vi "Add Key.vi"(6 "value":string, 8 "error in":errorcluster, 9 "key":string, 10 "section":string, 11 "Configuration File in":T1) -> (0 "error out":errorcluster, 3 "Configuration File out":T1)   [LabVIEW 2012, in "configlib.lvlib"]
uses:
  configlib.lvlib
  File Options.ctl
  Configuration File Definition.ctl
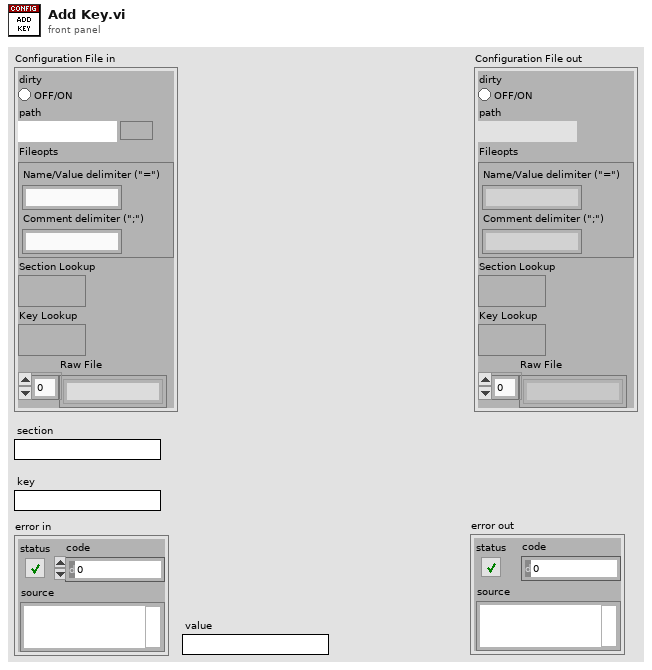
[diagram p1: front panel]
types:
  T1 = typedef "configlib.lvlib/Configuration File Definition.ctl" = cluster{"dirty":bool, "path":path, "Fileopts":T2, "Section Lookup":variant, "Key Lookup":variant, "Raw File":string[]}
  T2 = typedef "configlib.lvlib/File Options.ctl" = cluster{"Name/Value delimiter (\"=\")":string, "Comment delimiter (\";\")":string}
  T3 = typedef "configlib.lvlib/Section Definition.ctl" = cluster{"Keys":string[], "Segments":T4[]}
  T4 = typedef "configlib.lvlib/File Section.ctl" = cluster{"Line Number":i32, "Line Count":i32}
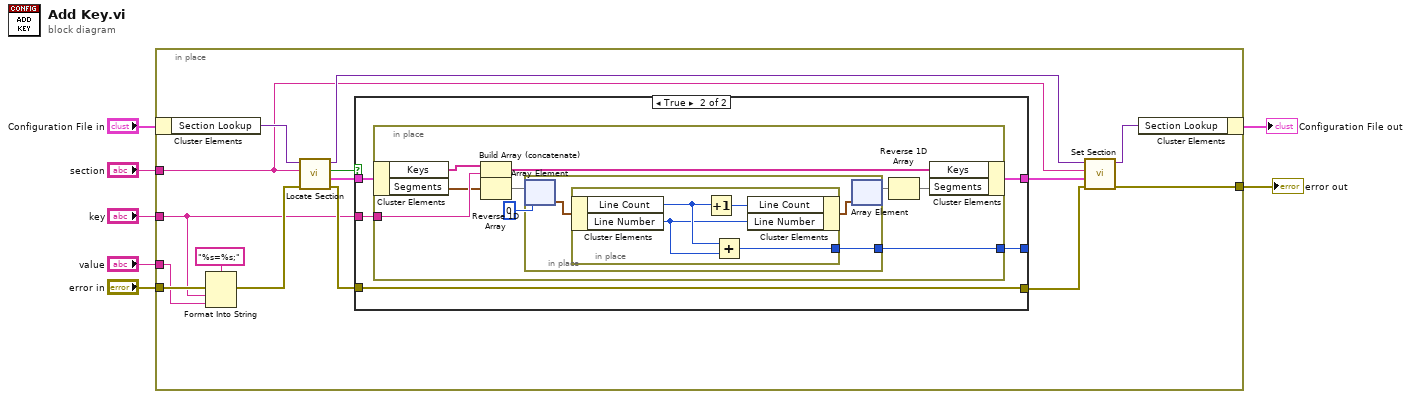
[diagram p0: block diagram]
diagram:
  n1 = in-place {
    in-place-border: "error in" -> [w12]
    in-place-border: "section" -> [w16]
    in-place-border: "key" -> [w8]
    in-place-border: "value" -> [w9]
    in-place-border: [w13] -> w1
    n2 = in-place-cluster #1("Configuration File in") -> ("Section Lookup"=w22:variant)
    n3 = Format Into String(format string="%s=%s;", error in=w12, w8, w9) -> (error out=w11:errorcluster)  [unwired: 1 in, 1 out]
    n4 = call "Locate Section.vi"("error in"=w11, "section"=w16, "key lookup"=w22) -> ("error out"=w19:errorcluster, "Section Definition"=w20:T3, "found?"=w21:bool, "key lookup out"=w18:variant)  [unwired: 5 in]
    n5 = case shown="True" w21 {
      tunnel: w20 -> [_ w26]
      tunnel: w19 -> [_ w24]
      tunnel: w8 -> [_ w27]
      tunnel: [_ w25] -> w17
      tunnel: [_ w24] -> w15
      tunnel: [_ w23] -> _
      frame False {
      }
      frame True {
        n6 = in-place {
          in-place-border: w27 -> [w36]
          in-place-border: [w28] -> w23
          n7 = in-place-cluster #2(w26) -> ("Keys"=w35:string[], "Segments"=w33:T4[])
          n8 = Build Array (concatenate)(w35, w36) -> (w34:string[])
          n9 = Reverse 1D Array(array=w33) -> (reversed array=w32:T4[])
          n10 = in-place {
            in-place-border: [w37] -> w28
            n11 = in-place-array #3(w32, 0) -> (w39:T4)
            n12 = in-place {
              in-place-border: [w40] -> w37
              n13 = in-place-cluster #4(w39) -> ("Line Count"=w43:i32, "Line Number"=w41:i32)
              n14 = Increment(x=w43) -> (x+1=w42:i32)
              n15 = Add(x=w43, y=w41) -> (x+y=w40:i32)
              n16 = in-place-cluster #4("Line Count"=w42, "Line Number"=w41) -> (w38:T4)
            }
            n17 = in-place-array #3(w38) -> (w30:T4[])  [unwired: 1 out]
          }
          n18 = Reverse 1D Array(array=w30) -> (reversed array=w29:T4[])
          n19 = in-place-cluster #2("Keys"=w34, "Segments"=w29) -> (w25:T3)
        }
      }
    }
    n20 = call "Set Section.vi"("error in"=w15, "Section Definition"=w17, "section"=w16, "key lookup"=w18) -> ("error out"=w13:errorcluster, "key lookup out"=w14:variant)  [unwired: 6 in]
    n21 = in-place-cluster #1("Section Lookup"=w14) -> (→"Configuration File out":T1)
  }
  "error out" <- w1
